vi "login to mtcdt to su root.vi"(6 "VISA resource name":refnum<visa-resource-name>, 7 "Passed so far?":bool=TRUE, 8 "error in (no error)":errorcluster) -> (0 "error out":errorcluster, 1 "read buffer 2":string, 2 "read buffer":string, 4 "VISA resource name out":refnum<visa-resource-name>, 5 "Passed?":bool)   [LabVIEW 2024]
uses:
  <vilib>/Instr/_visa.llb/VISA Configure Serial Port (Instr).vi
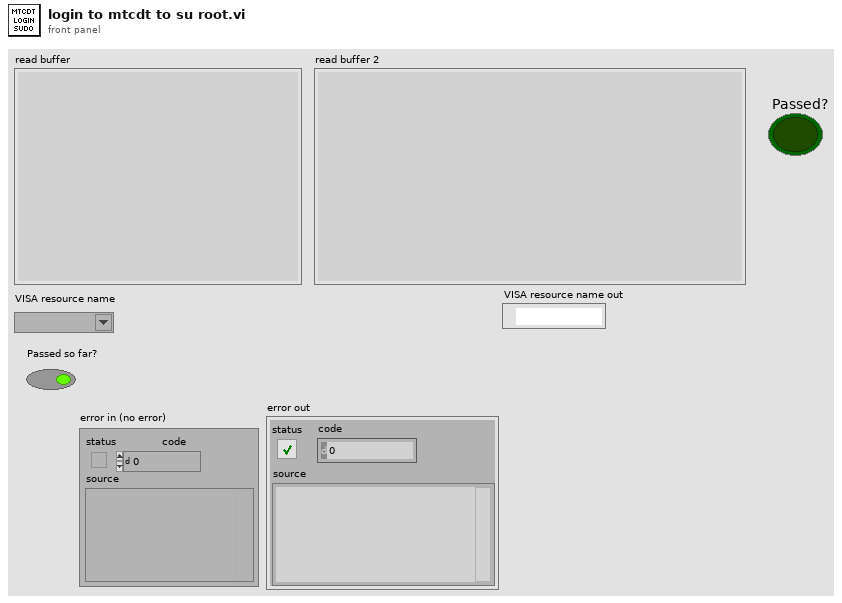
[diagram p1: front panel]
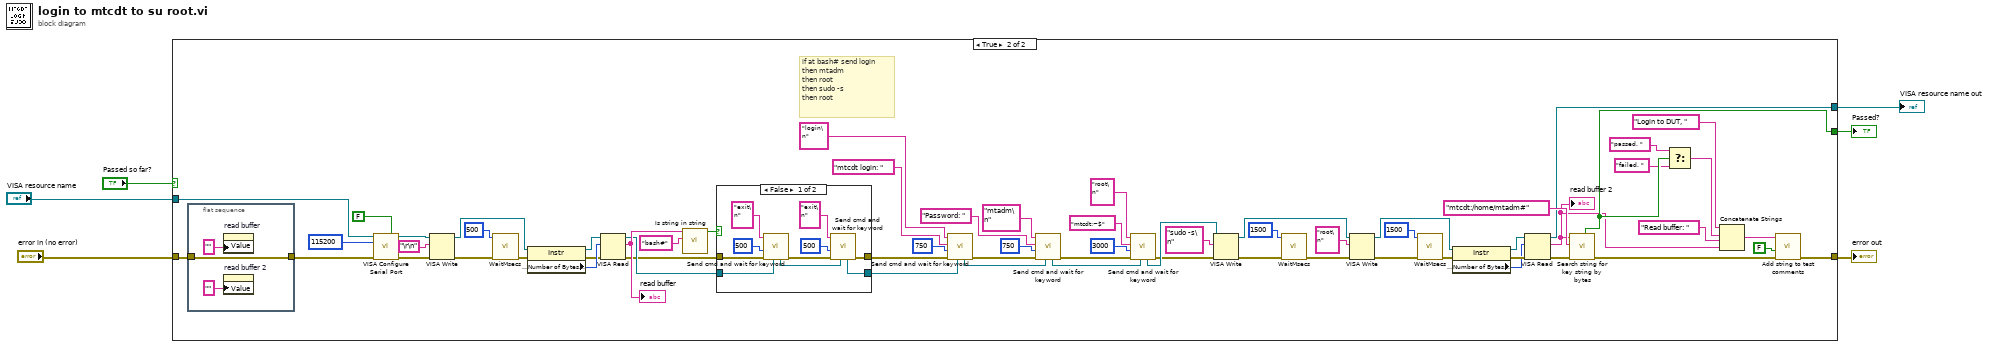
[diagram p0: block diagram]
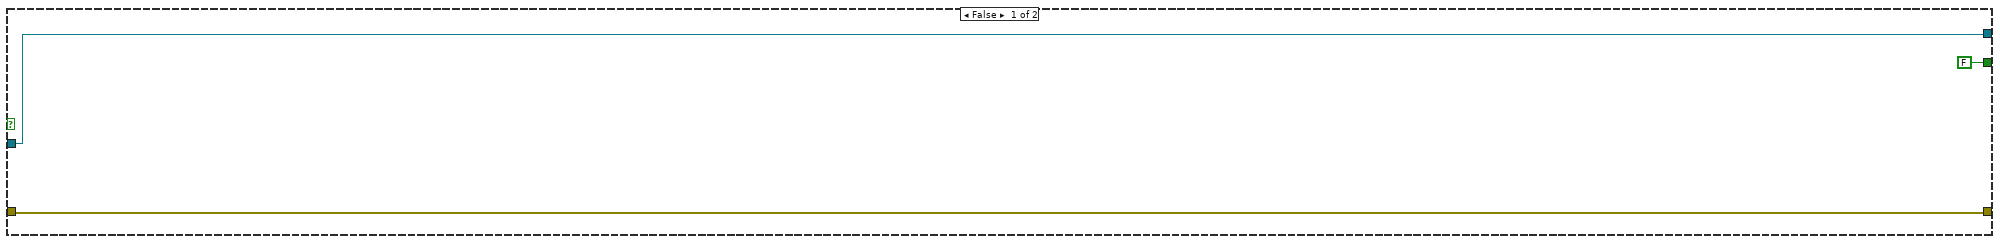
[diagram p2: hidden frame]
diagram:
  n1 = case shown="True" "Passed so far?" {
    tunnel: "error in (no error)" -> [w9 w59]
    tunnel: [w9 w52] -> w1
    tunnel: [FALSE ("Found match?") w50] -> w5
    tunnel: [w8 w55] -> w2
    tunnel: "VISA resource name" -> [w8 w54]
    frame False {
    }
    frame True {
      # "if at bash# send login\nthen mtadm\nthen root\nthen sudo -s\nthen root"
      n2 = flat-sequence {
        tunnel: w59 -> [w88]
        tunnel: [w88] -> w58
        frame #0 {
          n3 = property on="read buffer" class="Str"("Value"="" ("read buffer")) -> ()  [unwired: 2 in, 2 out]
          n4 = property on="read buffer 2" class="Str"("Value"="" ("read buffer 2")) -> ()  [unwired: 2 in, 2 out]
        }
      }
      n5 = call-poly "VISA Configure Serial Port"("VISA resource name"=w54, "Enable Termination\nChar (T)"=FALSE ("Enable Termination\nChar (T)"), "baud rate (9600)"=u32 115200, "error in (no error)"=w58) -> ("VISA resource name out"=w67:refnum<visa-resource-name>, "error out"=w68:errorcluster)  [unwired: 10 in]
      n6 = VISA Write(VISA resource name=w67, write buffer="\r\n", error in (no error)=w68) -> (VISA resource name out=w61:refnum<visa-resource-name>, error out=w73:errorcluster)  [unwired: 1 out]
      n7 = call "WaitMsecs.vi"("error in (no error)"=w73, "Wait Msecs"=u32 500) -> ("error out"=w62:errorcluster)  [unwired: 9 in]
      n8 = property class="Instr"(reference=w61, error in=w62) -> (reference out=w70:refnum<visa-resource-name>, error out=w71:errorcluster, "Serial Settings:Number of Bytes at Serial Port"=w72:u32)
      n9 = VISA Read(VISA resource name=w70, byte count=w72, error in (no error)=w71) -> (VISA resource name out=w42:refnum<visa-resource-name>, read buffer=w60:string, error out=w41:errorcluster)  [unwired: 1 out]
      "read buffer" <- w60
      n10 = call "Is string in string.vi"("Search for string"="bash#", "String buffer"=w60) -> ("In string?"=w38:bool)  [unwired: 8 in, 1 out]
      n11 = case shown="False" w38 {
        tunnel: w42 -> [w81 w85]
        tunnel: w41 -> [w80 w84]
        tunnel: [w75 w84] -> w40
        tunnel: [w74 w85] -> w39
        frame False {
          n12 = call "Send cmd and wait for keyword.vi"("VISA resource name"=w81, "error in (no error)"=w80, "Wait after"=u32 500 ("Wait Msecs"), "write buffer"="exit\n") -> ("error out"=w77:errorcluster, "VISA Refnum out"=w76:refnum<visa-resource-name>)  [unwired: 4 in, 2 out]
          n13 = call "Send cmd and wait for keyword.vi"("VISA resource name"=w76, "error in (no error)"=w77, "Wait after"=u32 500 ("Wait Msecs"), "write buffer"="exit\n") -> ("error out"=w75:errorcluster, "VISA Refnum out"=w74:refnum<visa-resource-name>)  [unwired: 4 in, 2 out]
        }
        frame True {
        }
      }
      n14 = call "Send cmd and wait for keyword.vi"("VISA resource name"=w39, "error in (no error)"=w40, "Wait after"=u32 750 ("Wait Msecs"), "Wait for"="mtcdt login: ", "write buffer"="login\n") -> ("error out"=w18:errorcluster, "VISA Refnum out"=w19:refnum<visa-resource-name>)  [unwired: 3 in, 2 out]
      n15 = call "Send cmd and wait for keyword.vi"("VISA resource name"=w19, "error in (no error)"=w18, "Wait after"=u32 750 ("Wait Msecs"), "Wait for"="Password: ", "write buffer"="mtadm\n") -> ("error out"=w14:errorcluster, "VISA Refnum out"=w12:refnum<visa-resource-name>)  [unwired: 3 in, 2 out]
      n16 = call "Send cmd and wait for keyword.vi"("VISA resource name"=w12, "error in (no error)"=w14, "Wait after"=u32 3000 ("Wait Msecs"), "Wait for"="mtcdt:~$", "write buffer"="root\n") -> ("error out"=w10:errorcluster, "VISA Refnum out"=w11:refnum<visa-resource-name>)  [unwired: 3 in, 2 out]
      n17 = VISA Write(VISA resource name=w11, write buffer="sudo -s\n", error in (no error)=w10) -> (VISA resource name out=w32:refnum<visa-resource-name>, error out=w33:errorcluster)  [unwired: 1 out]
      n18 = call "WaitMsecs.vi"("error in (no error)"=w33, "Wait Msecs"=u32 1500) -> ("error out"=w35:errorcluster)  [unwired: 9 in]
      n19 = VISA Write(VISA resource name=w32, write buffer="root\n", error in (no error)=w35) -> (VISA resource name out=w28:refnum<visa-resource-name>, error out=w26:errorcluster)  [unwired: 1 out]
      n20 = call "WaitMsecs.vi"("error in (no error)"=w26, "Wait Msecs"=u32 1500) -> ("error out"=w25:errorcluster)  [unwired: 9 in]
      n21 = property class="Instr"(reference=w28, error in=w25) -> (reference out=w31:refnum<visa-resource-name>, error out=w30:errorcluster, "Serial Settings:Number of Bytes at Serial Port"=w29:u32)
      n22 = VISA Read(VISA resource name=w31, byte count=w29, error in (no error)=w30) -> (VISA resource name out=w55:refnum<visa-resource-name>, read buffer=w45:string, error out=w56:errorcluster)  [unwired: 1 out]
      "read buffer 2" <- w45
      n23 = call "Search string for key string by bytes.vi"("error in (no error)"=w56, "Search for string"="mtcdt:/home/mtadm#", "String"=w45) -> ("error out"=w53:errorcluster, "Found match?"=w50:bool)  [unwired: 4 in, 3 out]
      n24 = Select(t="passed. ", s=w50, f="failed. ") -> (s? t:f=w47:string)
      n25 = Concatenate Strings("Login to DUT, " ("string"), w47, "Read buffer: " ("string"), w45) -> (w44:string)
      n26 = call "Add string to test comments.vi"("error in (no error)"=w53, "New Section (y)?"=FALSE, "Comments"=w44) -> ("error out"=w52:errorcluster)  [unwired: 7 in, 1 out]
    }
  }
  "Passed?" <- w5
  "error out" <- w1
  "VISA resource name out" <- w2
